vi "WebView2 Updater.vi"() -> ()   [LabVIEW 2020, in "WebView2 Updater.lvclass"]
uses:
  WebView2 Updater.lvclass
  WebView2 Updater.lvclass/WebView2 Updater.ctl
panel:
  in  "Tab Control":T1(tab)
  out "Installed version":string
  in  "Selected Version":string(combo)
  in  "Prerelease?":bool
  in  "Older?":bool
  out "Installed version 2":string caption="Installed"
  out "Step":string
  out "Compiled":bool
  out "Relinked":bool
  out "Downloaded":bool
  out "URL":string
  out "Build Date":timestamp format="%<%x %.3X>T"
  out "Copied":bool
  out "Unzipped":bool
  out "New Version":string
  in  "Skip":bool
  in  "Check Updates":bool
  # "Check for WebView2 Assembly updates?"
  # "Select version to download and install.\nSee link for version details."
  # "Include"
  # "https://www.nuget.org/packages/Microsoft.Web.WebView2"
  # "Update complete. New installed version:"
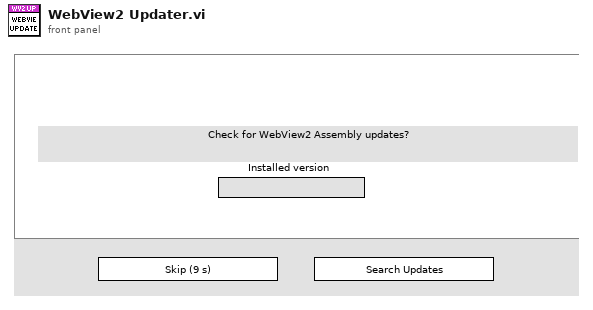
[diagram p1: front panel]
types:
  T1 = enum32{"Start", "Versions", "Install", "Complete"}
  T2 = enum16{"Exit", "Init", "Get Installed Version", "Start", "List Versions", "Filter Versions", "Select Version", "Download Package", "Update Package", "Relink Nodes", "Mass Compile", "Complete"}
  T3 = enum32{"Invalid", "Standard", "Closed", "Hidden", "Minimized", "Maximized"}
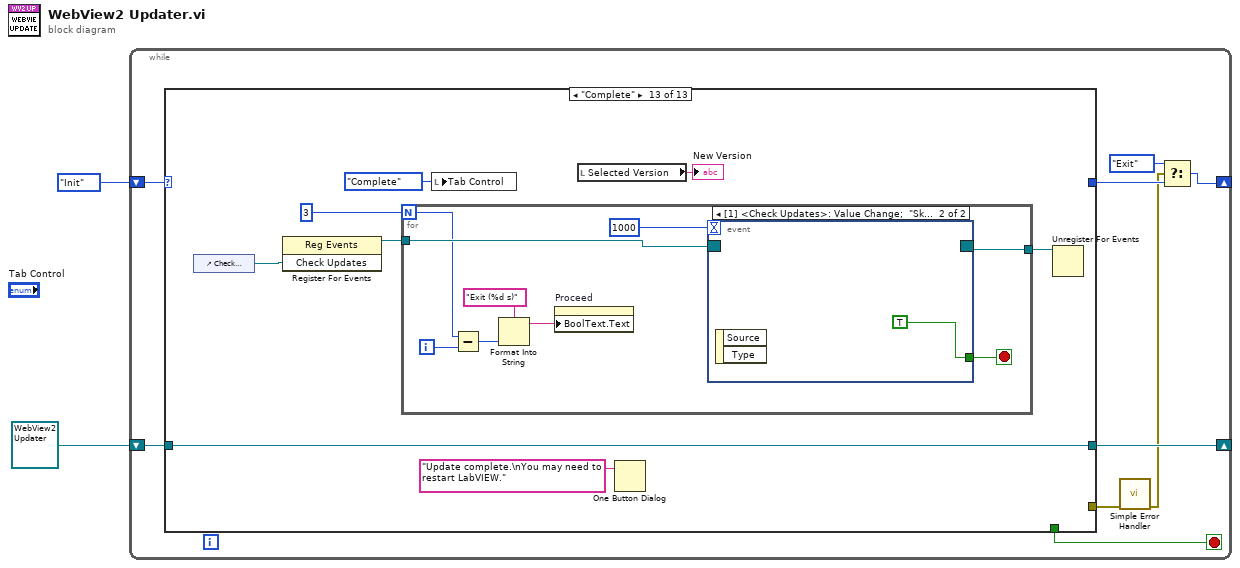
[diagram p0: block diagram]
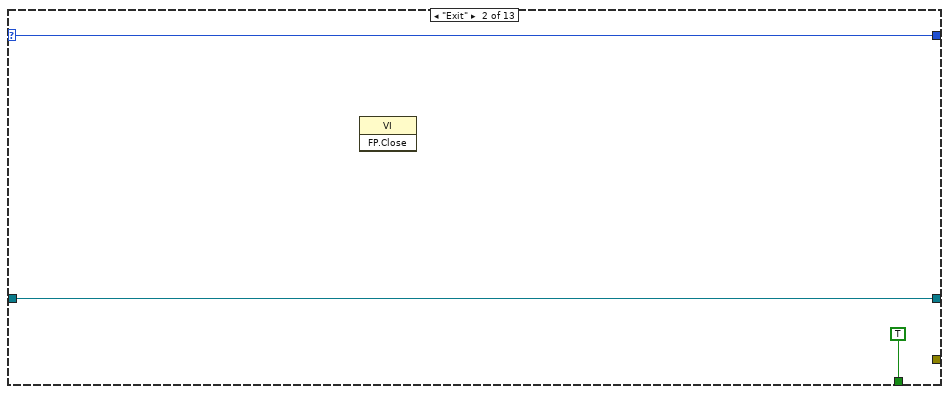
[diagram p4: hidden frame]
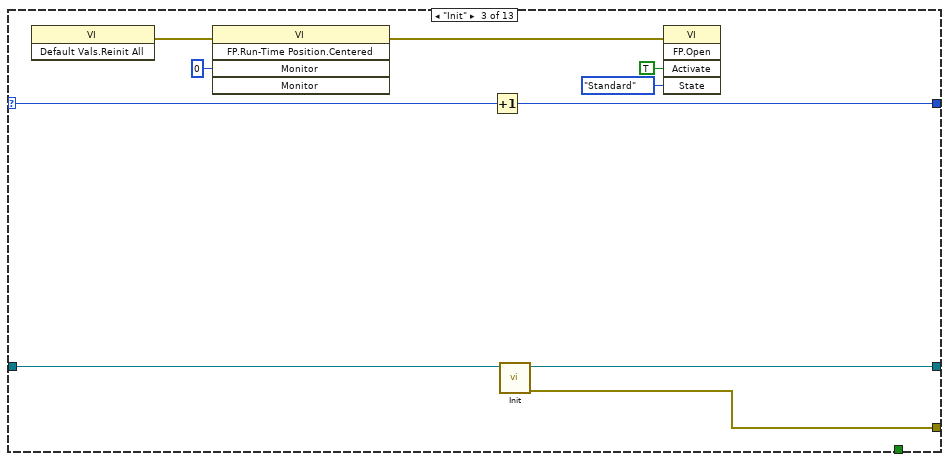
[diagram p5: hidden frame]
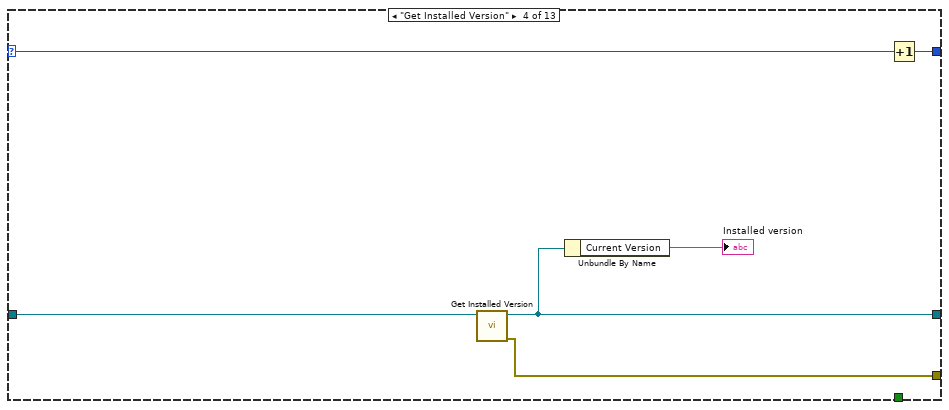
[diagram p6: hidden frame]
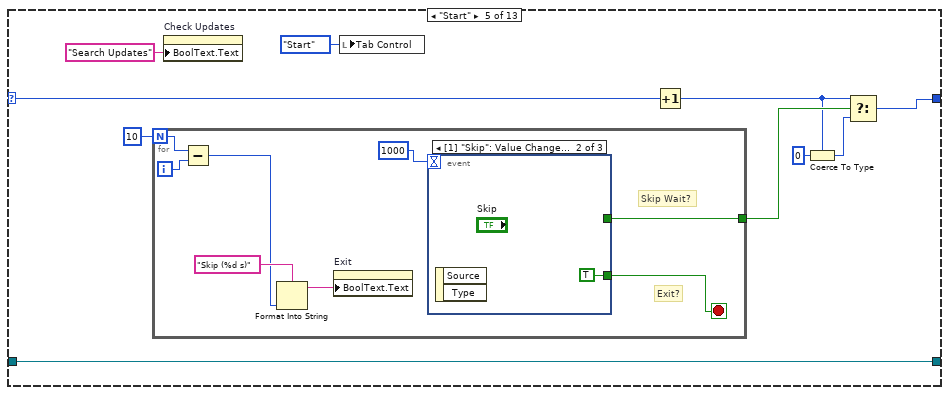
[diagram p7: hidden frame]
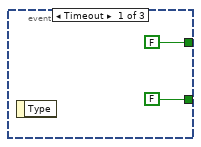
[diagram p8: hidden frame]
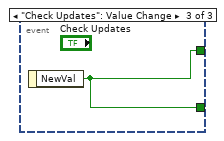
[diagram p9: hidden frame]
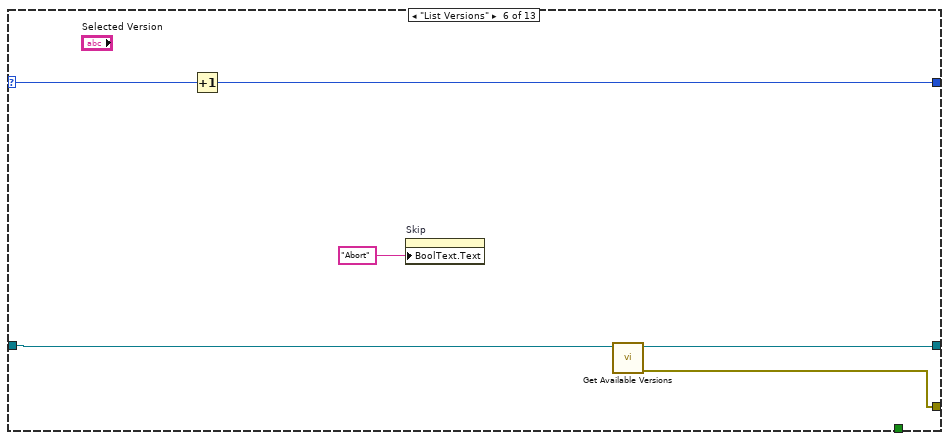
[diagram p10: hidden frame]
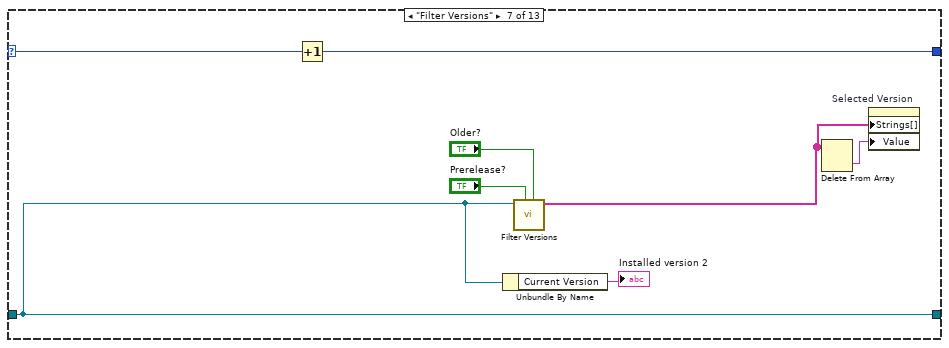
[diagram p11: hidden frame]
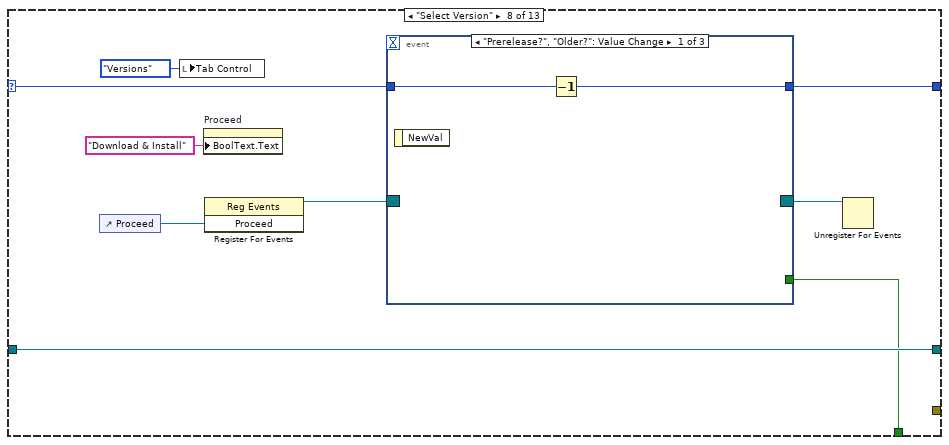
[diagram p12: hidden frame]
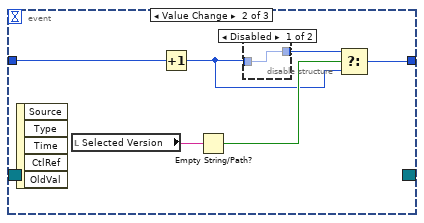
[diagram p13: hidden frame]
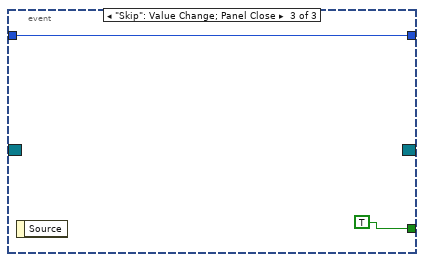
[diagram p15: hidden frame]
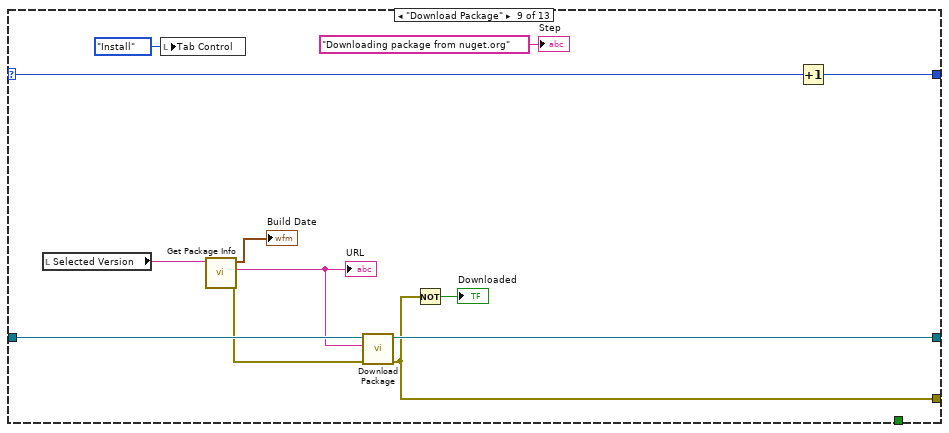
[diagram p16: hidden frame]
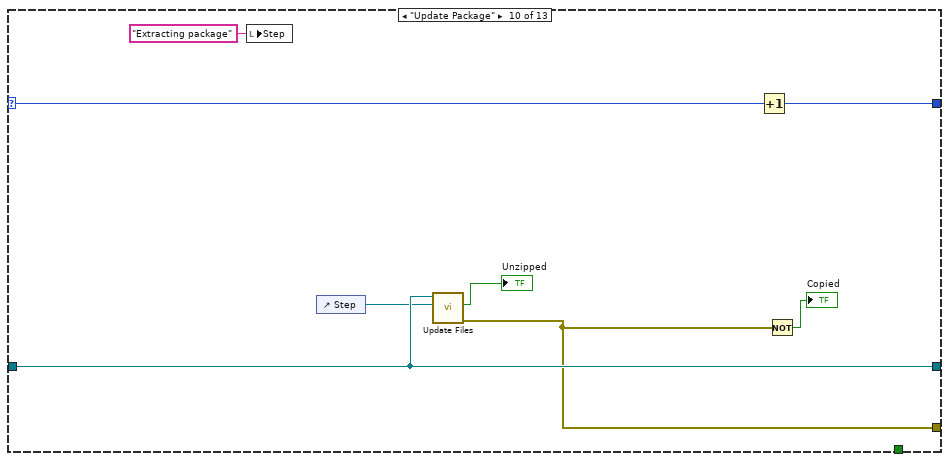
[diagram p17: hidden frame]
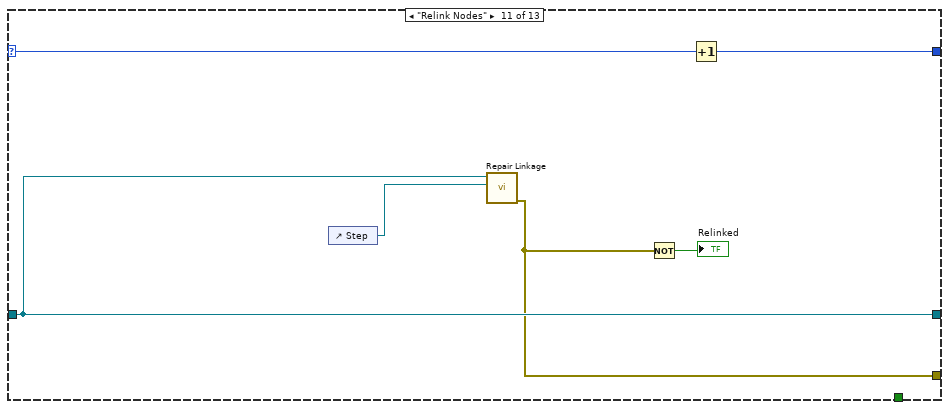
[diagram p18: hidden frame]
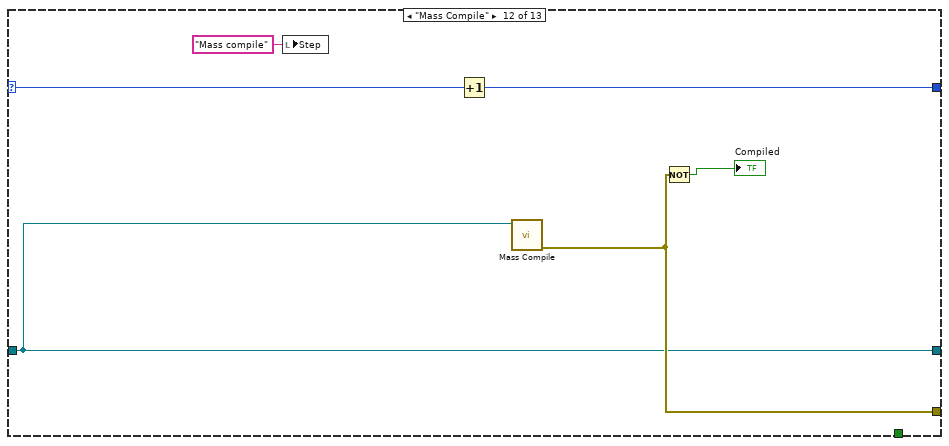
[diagram p19: hidden frame]
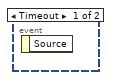
[diagram p20: hidden frame]
diagram:
  n1 = while {
    shift-right: [w10] -> _
    shift-left: refnum<class "WebView2 Updater.lvclass"> refnum ("WebView2 Updater.lvclass") -> [w11]
    shift-right: [w5] -> _
    shift-left: T2."Init" -> [w7]
    stop <- w9 stop-if-true
    n2 = case shown="\"Complete\"" w7 {
      selector: w7 -> [w12 w16 w27 w33 w41 w60 w68 w77 w101 w107 w116 w122 _]
      tunnel: w11 -> [w14 w18 w20 w34 w44 w62 w64 w79 w102 w110 w114 w117 w130]
      tunnel: [w14 w18 w28 w30 w44 w61 w64 w79 w99 w110 w114 w117 w130] -> w10
      tunnel: [w13 w16 w26 w32 w40 w59 w67 w78 w100 w106 w115 w121 _] -> w8
      tunnel: [_ TRUE _ _ _ _ _ w73 _ _ _ _ _] -> w9
      tunnel: [_ _ w25 w31 _ w58 _ _ w92 w108 w111 w120 _] -> w6
      frame Default {
        n3 = disable-structure shown="Disabled" {
          disable-tunnel: [w15 _] -> w13
          disable-tunnel: w12 -> [w15 _]
          frame Disabled {
          }
          frame Enabled {
          }
        }
      }
      frame "Exit" {
        n4 = invoke class="VI" method="FP.Close"() -> ()  [unwired: 3 in, 3 out]
      }
      frame "Init" {
        n5 = invoke class="VI" method="Default Vals.Reinit All"() -> (error out=w19:errorcluster)  [unwired: 3 in, 2 out]
        n6 = invoke class="VI" method="FP.Run-Time Position.Centered"(error in=w19, "Monitor"=i16 0) -> (error out=w23:errorcluster)  [unwired: 3 in, 4 out]
        n7 = Increment(x=w27) -> (x+1=w26:T2)
        n8 = call "Init.vi"("WebView2 Updater in"=w20) -> ("error out"=w25:errorcluster, "WebView2 Updater out"=w28:refnum<class "WebView2 Updater.lvclass">)  [unwired: 9 in]
        n9 = invoke class="VI" method="FP.Open"(error in=w23, "Activate"=TRUE ("Activate?"), "State"=T3."Standard") -> ()  [unwired: 2 in, 5 out]
      }
      frame "Get Installed Version" {
        n10 = call "Get Installed Version.vi"("WebView2 Updater in"=w34) -> ("error out"=w31:errorcluster, "WebView2 Updater out"=w30:refnum<class "WebView2 Updater.lvclass">)  [unwired: 9 in]
        n11 = Unbundle By Name(w30) -> ("Current Version"=→"Installed version":string)
        n12 = Increment(x=w33) -> (x+1=w32:T2)
      }
      frame "Start" {
        n13 = for {
          N: 10 -> [w51]
          tunnel: [w45] -> w42
          i -> [w50]
          stop <- w46 stop-if-true
          # "Skip Wait?"
          # "Exit?"
          n14 = Subtract(x=w51, y=w50) -> (x-y=w48:i32)
          n15 = Format Into String(format string="Skip (%d s)", w48) -> (resulting string=w47:string)  [unwired: 2 in, 1 out]
          n16 = property on="Exit" class="Bool"("BoolText.Text"=w47) -> ()  [unwired: 2 in, 2 out]
          n17 = event shown="[1] \"Skip\": Value Change;  Panel Close" {
            selector: _ -> [_ _ _]
            dyn-events: _ -> [_ _ _]
            timeout: 1000 -> [_ _ _]
            tunnel: [FALSE TRUE ("NewVal") w56] -> w46
            tunnel: [FALSE _ w56] -> w45
            event Timeout {
              n18 = event-data() -> ()  [unwired: 1 in, 1 out]
            }
            event "Skip": Value Change; Panel Close {
              n19 = event-data() -> ()  [unwired: 1 in, 2 out]
            }
            event "Check Updates": Value Change {
              n20 = event-data() -> ("NewVal"=w56:bool)  [unwired: 1 in]
            }
          }
        }
        n21 = property on="Check Updates" class="Bool"("BoolText.Text"="Search Updates" ("Boolean Text.Text")) -> ()  [unwired: 2 in, 2 out]
        n22 = local write "Tab Control"(T1."Start" ("Tab Control")) -> ()
        n23 = Increment(x=w41) -> (x+1=w37:T2)
        n24 = Coerce To Type(0:0, 1:w37) -> (2:w38:T2)
        n25 = Select(t=w37, s=w42, f=w38) -> (s? t:f=w40:T2)
      }
      frame "List Versions" {
        n26 = Increment(x=w60) -> (x+1=w59:T2)
        n27 = property on="Skip" class="Bool"("BoolText.Text"="Abort" ("Boolean Text.Text")) -> ()  [unwired: 2 in, 2 out]
        n28 = call "Get Available Versions.vi"("WebView2 Updater in"=w62) -> ("error out"=w58:errorcluster, "WebView2 Updater out"=w61:refnum<class "WebView2 Updater.lvclass">)  [unwired: 9 in]
      }
      frame "Filter Versions" {
        n29 = Increment(x=w68) -> (x+1=w67:T2)
        n30 = Unbundle By Name(w64) -> ("Current Version"=→"Installed version 2":string)
        n31 = call "Filter Versions.vi"("Older?"="Older?", "Prerelease?"="Prerelease?", "WebView2 Updater in"=w64) -> ("Array"=w69:string[])  [unwired: 8 in]
        n32 = Delete From Array(array=w69) -> (deleted portion=w70:string)  [unwired: 2 in, 1 out]
        n33 = property on="Selected Version" class="CmbBox"("Strings[]"=w69, "Value"=w70) -> ()  [unwired: 2 in, 2 out]
      }
      frame "Select Version" {
        n34 = control-ref of="Proceed"() -> (w76:refnum<vi>)
        n35 = local write "Tab Control"(T1."Versions" ("Tab Control")) -> ()
        n36 = property on="Proceed" class="Bool"("BoolText.Text"="Download & Install" ("Boolean Text.Text")) -> ()  [unwired: 2 in, 2 out]
        n37 = register-events(w76) -> (reference out=w75:refnum<event-registration>)  [unwired: 2 in, 1 out]
        n38 = event shown="[0] \"Prerelease?\", \"Older?\": Value Change" {
          selector: w75 -> [_ _ _]
          dyn-events: [_ _ _] -> w74
          timeout: _ -> [_ _ _]
          tunnel: [w80 w85 w90] -> w78
          tunnel: w77 -> [w81 w87 w90]
          tunnel: [_ _ TRUE] -> w73
          event "Prerelease?", "Older?": Value Change {
            n39 = event-data() -> ()  [unwired: 1 in, 1 out]
            n40 = Decrement(x=w81) -> (x-1=w80:T2)
          }
          event Value Change {
            n41 = event-data() -> ()  [unwired: 1 in, 5 out]
            n42 = local read "Selected Version"() -> (w86:string)
            n43 = Increment(x=w87) -> (x+1=w82:T2)
            n44 = Empty String/Path?(string/path=w86) -> (empty?=w84:bool)
            n45 = disable-structure shown="Disabled" {
              disable-tunnel: [w88 _] -> w83
              disable-tunnel: w82 -> [w88 _]
              frame Disabled {
              }
              frame Enabled {
              }
            }
            n46 = Select(t=w83, s=w84, f=w82) -> (s? t:f=w85:T2)
          }
          event "Skip": Value Change; Panel Close {
            n47 = event-data() -> ()  [unwired: 1 in, 1 out]
          }
        }
        n48 = Unregister For Events(event registration refnum=w74) -> ()  [unwired: 1 in, 1 out]
      }
      frame "Download Package" {
        n49 = local read "Selected Version"() -> (w96:string)
        n50 = local write "Tab Control"(enum32{"Start", "Versions", "Install"}."Install" ("Tab Control")) -> ()
        n51 = call "Get Package Info.vi"("Selected Version"=w96) -> ("error out"=w93:errorcluster, "URL"=w94:string, "Build Date"=→"Build Date":timestamp)  [unwired: 8 in]
        "URL" <- w94
        n52 = call "Download Package.vi"("error in (no error)"=w93, "URL"=w94, "WebView2 Updater in"=w102) -> ("error out"=w92:errorcluster, "WebView2 Updater out"=w99:refnum<class "WebView2 Updater.lvclass">)  [unwired: 7 in]
        n53 = Not(x=w92) -> (.not. x?=→"Downloaded":bool)
        n54 = Increment(x=w101) -> (x+1=w100:T2)
        "Step" <- "Downloading package from nuget.org" ("Step")
      }
      frame "Update Package" {
        n55 = local write "Step"("Extracting package" ("Step")) -> ()
        n56 = control-ref of="Step"() -> (w104:refnum<vi>)
        n57 = call "Update Files.vi"("Step"=w104, "WebView2 Updater in"=w110) -> ("error out"=w108:errorcluster, "Unzipped"=→"Unzipped":bool)  [unwired: 8 in]
        n58 = Increment(x=w107) -> (x+1=w106:T2)
        n59 = Not(x=w108) -> (.not. x?=→"Copied":bool)
      }
      frame "Relink Nodes" {
        n60 = control-ref of="Step"() -> (w112:refnum<vi>)
        n61 = call "Repair Linkage.vi"("Status"=w112, "WebView2 Updater in"=w114) -> ("error out"=w111:errorcluster)  [unwired: 9 in]
        n62 = Not(x=w111) -> (.not. x?=→"Relinked":bool)
        n63 = Increment(x=w116) -> (x+1=w115:T2)
      }
      frame "Mass Compile" {
        n64 = local write "Step"("Mass compile" ("Step")) -> ()
        n65 = Increment(x=w122) -> (x+1=w121:T2)
        n66 = call "Mass Compile.vi"("WebView2 Updater in"=w117) -> ("error out"=w120:errorcluster)  [unwired: 10 in]
        n67 = Not(x=w120) -> (.not. x?=→"Compiled":bool)
      }
      frame "Complete" {
        n68 = control-ref of="Check Updates"() -> (w126:refnum<vi>)
        n69 = register-events(w126) -> (reference out=w125:refnum<event-registration>)  [unwired: 2 in, 1 out]
        n70 = for {
          N: 3 -> [w136]
          tunnel: w125 -> [w138]
          tunnel: [w137] -> w124
          i -> [w135]
          stop <- w131 stop-if-true
          n71 = Subtract(x=w136, y=w135) -> (x-y=w134:i32)
          n72 = Format Into String(format string="Exit (%d s)" ("Boolean Text.Text"), w134) -> (resulting string=w132:string)  [unwired: 2 in, 1 out]
          n73 = property on="Proceed" class="Bool"("BoolText.Text"=w132) -> ()  [unwired: 2 in, 2 out]
          n74 = event shown="[1] <Check Updates>: Value Change;  \"Skip\": Value Change;  Panel Close" {
            selector: w138 -> [_ _]
            dyn-events: [_ _] -> w137
            timeout: 1000 -> [_ _]
            tunnel: [_ TRUE] -> w131
            event Timeout {
              n75 = event-data() -> ()  [unwired: 1 in, 1 out]
            }
            event "Skip": Value Change; Panel Close {
              n76 = event-data() -> ()  [unwired: 1 in, 2 out]
            }
          }
        }
        n77 = local write "Tab Control"(T1."Complete" ("Tab Control")) -> ()
        n78 = local read "Selected Version"() -> (→"New Version":string)
        n79 = One Button Dialog(message="Update complete.\nYou may need to restart LabVIEW.") -> ()  [unwired: 1 in, 1 out]
        n80 = Unregister For Events(event registration refnum=w124) -> ()  [unwired: 1 in, 1 out]
      }
    }
    n81 = call <vilib>:"Simple Error Handler.vi"("error in (no error)"=w6) -> ("error out"=w4:errorcluster)  [unwired: 4 in, 4 out]
    n82 = Select(t=T2."Exit", s=w4, f=w8) -> (s? t:f=w5:T2)
  }
